vi "Assert.vi"(4 "Variable Y":variant, 6 "Variable X":variant, 11 "Assert Equal in":refnum<class "Assert Less.lvclass">) -> (2 "Assert?":bool)   [LabVIEW 2019, in "Run Time Assertions.lvlib" / "Assert Less.lvclass"]
uses:
  <vilib>/gpm_packages/@cs/run-time-assertions/Source/Assert Less/Assert Less.lvclass
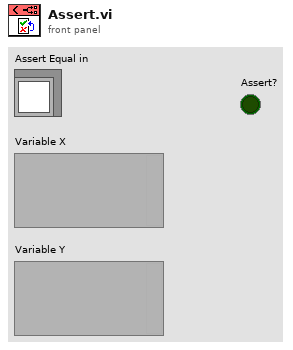
[diagram p1: front panel]
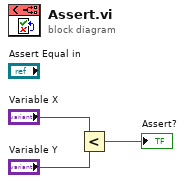
[diagram p0: block diagram]
diagram:
  n1 = Less?(x="Variable X", y="Variable Y") -> (x < y?=→"Assert?":bool)
